vi "Create Read Event.vi"(8 "error in":errorcluster, 11 "Read Event in":refnum<class "Read Event.lvclass">) -> (0 "error out":errorcluster, 3 "Read Event out":refnum<class "Read Event.lvclass">)   [LabVIEW 2019, in "PCANBasic.lvlib" / "Read Event.lvclass"]
doc: "If the function succeeds, the return value is a handle to the event object."
uses:
  Read Event.lvclass
  Read Event.lvclass/Read Event.ctl
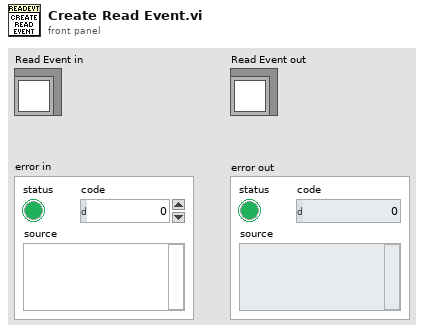
[diagram p1: front panel]
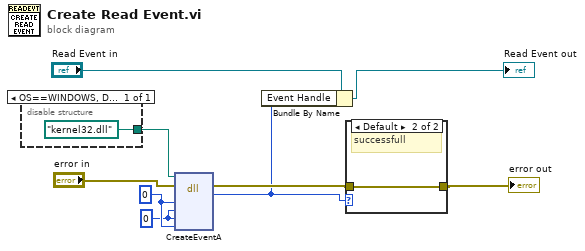
[diagram p0: block diagram]
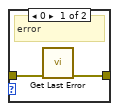
[diagram p2: hidden frame]
diagram:
  w7 = 0 ("lpName")
  w8 = u64 0 ("lpName")
  n1 = disable-structure shown="OS==WINDOWS, Default" {
    disable-tunnel: [path "kernel32.dll" ("path in")] -> w9
    frame condition #0 (active) {
    }
  }
  n2 = dll-call lib="?" fn="CreateEventA"(path in=w9, error in="error in", "lpEventAttributes"=w8, "bManualReset"=w7, "bInitialState"=w7, "lpName"=w8) -> (error out=w4:errorcluster, "hdlEvent"=w1:u64)  [unwired: 5 in, 1 out]
  n3 = Bundle By Name(cluster="Read Event in", "Event Handle"=w1) -> (→"Read Event out":refnum<class "Read Event.lvclass">)
  n4 = case "success?" shown="Default" w1 {
    tunnel: w4 -> [w12 w13]
    tunnel: [w11 w13] -> w5
    frame 0 {
      # "error"
      n5 = call "Get Last Error.vi"("error in"=w12) -> ("error out"=w11:errorcluster)  [unwired: 10 in]
    }
    frame Default {
      # "successfull"
    }
  }
  "error out" <- w5
